vi "Detect Color.vi"() -> ()   [LabVIEW 2016]
uses:
  <vilib>/NXT/Block Support/NXT_InputPort.ctl
  <vilib>/NXT/Subs/ColorSensorColors.ctl
  <vilib>/NXT/Block Support/NXT_OutputPort.ctl
  <vilib>/NXT/Dual Mode Library/Sensors/EV3_Color_Color.vi
  <vilib>/NXT/NXTIO Xnodes/NXTIONodeSubVIs/NXTMoveMotors.vi
  <vilib>/NXT/Dual Mode Library/Waits/Wait_Num.vi
  <vilib>/NXT/NXTIO Xnodes/NXTIONodeSubVIs/LEGOStopAllMotors.vi
  <vilib>/NXT/Subs/LVHSConnector.ctl
  <vilib>/NXT/NXTIO Xnodes/AddressXNode/NXTIOAddress.xnode
  <vilib>/NXT/NXTIO Xnodes/NXTIOXNode/NXTIO.xnode
  <vilib>/NXT/LegoClasses/BrickReference/BrickReference.lvclass
panel:
  in  "stop":bool
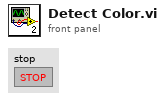
[diagram p1: front panel]
types:
  T1 = typedef "ColorSensorColors.ctl" = enum16{"No Color", "Black", "Blue", "Green", "Yellow", "Red", "White", "Brown"}
  T2 = typedef "NXT_InputPort.ctl" = u32
  T3 = typedef "NXT_OutputPort.ctl" = u8
  T4 = typedef "LVHSConnector.ctl" = refnum<class "BrickReference.lvclass">
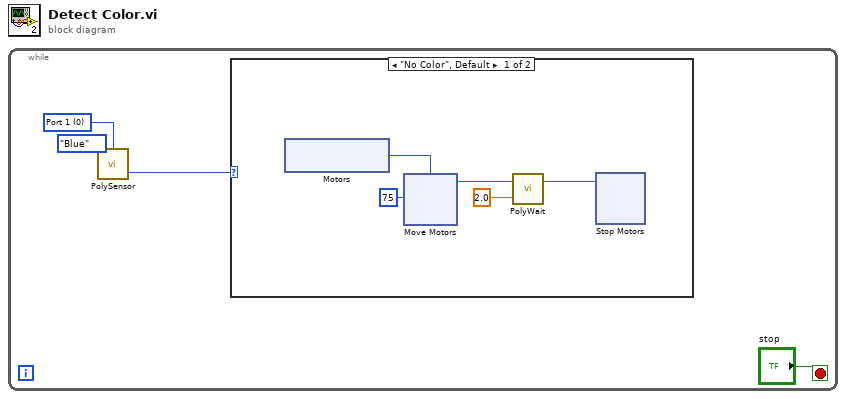
[diagram p0: block diagram]
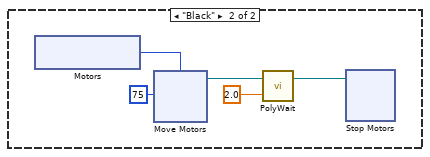
[diagram p2: hidden frame]
diagram:
  n1 = while {
    stop <- "stop" stop-if-true
    (unwired) ColorSensorColors."Blue" ("Detected Color")
    w3 = T2 0 items=["Port 1", "Port 2", "Port 3", "Port 4"] ("Port (Port 1)")
    n2 = call-poly <vilib>:"PolySensor.vi"("Port (Port 1)"=w3) -> ("Detected Color"=w2:T1)  [unwired: 2 in, 1 out]
    n3 = case shown="\"No Color\", Default" w2 {
      frame "No Color", Default {
        n4 = xnode "Motors"() -> ("Motor"=w7:T3)
        n5 = xnode "Move Motors"("Power/Speed 1"=i8 75, "Motors"=w7) -> ("NXT/EV3"=w5:T4)  [unwired: 1 in]
        n6 = call-poly <vilib>:"PolyWait.vi"("Time (1 sec)"=sgl 2.0, "NXT/EV3"=w5) -> ("NXT/EV3"=w4:T4)  [unwired: 2 in]
        n7 = xnode "Stop Motors"("NXT/EV3"=w4) -> ()  [unwired: 1 in, 1 out]
      }
      frame "Black" {
        n8 = xnode "Motors"() -> ("Motor"=w21:T3)
        n9 = xnode "Move Motors"("Power/Speed 1"=i8 75, "Motors"=w21) -> ("NXT/EV3"=w23:T4)  [unwired: 1 in]
        n10 = call-poly <vilib>:"PolyWait.vi"("Time (1 sec)"=sgl 2.0, "NXT/EV3"=w23) -> ("NXT/EV3"=w24:T4)  [unwired: 2 in]
        n11 = xnode "Stop Motors"("NXT/EV3"=w24) -> ()  [unwired: 1 in, 1 out]
      }
    }
  }
